vi "Primite_Lottery.vi"   [LabVIEW 2020]
uses:
  <vilib>/Utility/file.llb/Write Delimited Spreadsheet (DBL).vi
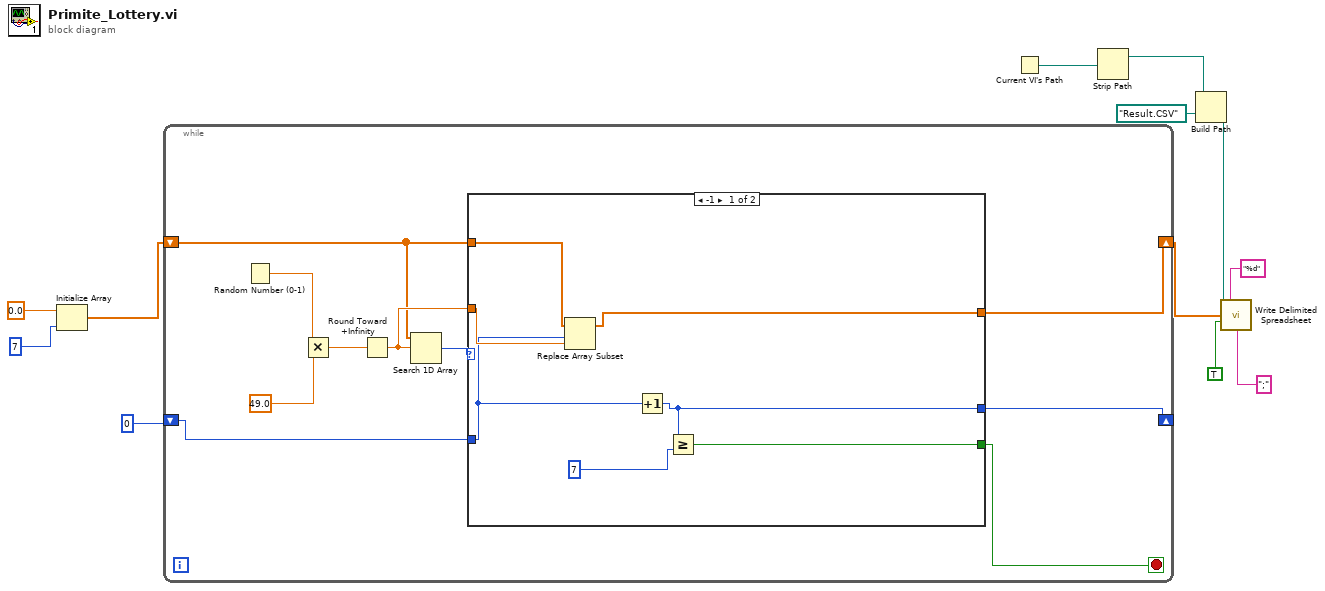
[diagram p0: block diagram]
diagram:
  n1 = Initialize Array(0.0, 7) -> (w9:dbl[])
  n2 = while {
    shift-right: [w14] -> w7
    shift-left: w9 -> [w17]
    shift-right: [w15] -> _
    shift-left: 0 -> [w19]
    stop <- w16 stop-if-true
    n3 = Random Number (0-1)() -> (number: 0 to 1=w22:dbl)
    n4 = Multiply(x=w22, y=49.0) -> (x*y=w20:dbl)
    n5 = Round Toward +Infinity(x=w20) -> (ceil(x): smallest int >= x=w18:dbl)
    n6 = Search 1D Array(1D array=w17, element=w18) -> (index of element=w13:i32)  [unwired: 1 in]
    n7 = case shown="-1" w13 {
      tunnel: w17 -> [w29 _]
      tunnel: [w28 _] -> w14
      tunnel: w19 -> [w23 _]
      tunnel: w18 -> [w27 _]
      tunnel: [w25 _] -> w15
      tunnel: [w24 _] -> w16
      frame -1 {
        n8 = Replace Array Subset(array=w29, new element=w27, index=w23) -> (w28:dbl[])
        n9 = Increment(x=w23) -> (x+1=w25:i32)
        n10 = Greater Or Equal?(x=w25, y=7) -> (x >= y?=w24:bool)
      }
      frame 0, Default {
      }
    }
  }
  n11 = Current VI's Path() -> (path=w4:path)
  n12 = Strip Path(path=w4) -> (stripped path=w5:path)  [unwired: 1 out]
  n13 = Build Path(base path=w5, name or relative path=path "Result.CSV") -> (appended path=w6:path)
  n14 = call-poly <vilib>:"Write Delimited Spreadsheet.vi"("file path (dialog if empty)"=w6, "format (%.3f)"="%d", "1D data"=w7, "append to file? (new file:F)"=TRUE, "delimiter (\\t)"=";") -> ()  [unwired: 9 in, 2 out]
